vi "InitCursor.vi"(8 "error in (no error)":errorcluster, 11 "Menu in":refnum<class "Menu.lvclass">) -> (0 "error out":errorcluster, 3 "Menu out":refnum<class "Menu.lvclass">)   [LabVIEW 2019, in "RT_Game.lvlib" / "Menu.lvclass"]
uses:
  Menu.lvclass
  C:/Users/FreshBob/Dropbox/VIs/myRIO_GameConsole/RT/RT_Game/Game/Game.lvclass
  Cursor/Cursor.lvclass
  C:/Users/FreshBob/Dropbox/VIs/myRIO_GameConsole/RT/RT_Game/GameObject/GameObject.lvclass
  C:/Users/FreshBob/Dropbox/VIs/myRIO_GameConsole/RT/RT_Game/RT_Sprite/RT_Sprite.lvclass
  Game/Coordinate.ctl
  Menu.lvclass/Menu.ctl
  Cursor/Cursor.lvclass/Cursor.ctl
  GameObject/GameObject.lvclass/GameObject.ctl
  Game/Game.lvclass/Game.ctl
  Cursor/Write Positions.vi
  Cursor/Write selection.vi
  Cursor/Write speed.vi
  GameObject/Write IsActive.vi
  Cursor/Write Wrap.vi
  Game/Write Sprite1.vi
  Game/Game.lvclass
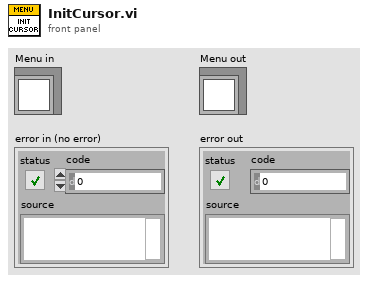
[diagram p1: front panel]
types:
  T1 = typedef "RT_Game.lvlib/Game.lvclass/Coordinate.ctl" = cluster{"x":dbl, "y":dbl}
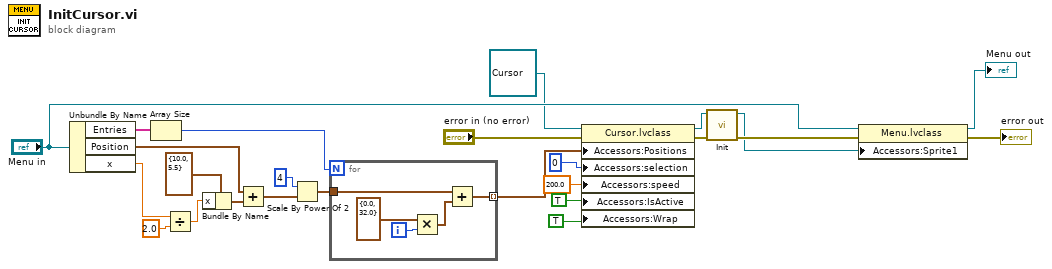
[diagram p0: block diagram]
diagram:
  n1 = Unbundle By Name("Menu in") -> ("Entries"=w10:string[], "Position"=w11:T1, "x"=w14:dbl)
  n2 = Array Size(array=w10) -> (size(s)=w18:i32)
  n3 = Divide(x=w14, y=2.0) -> (x/y=w16:dbl)
  n4 = Bundle By Name(cluster=T1 {"x"=10.0, "y"=5.5} ("y"), "x"=w16) -> (w13:T1)
  n5 = Add(x=w11, y=w13) -> (x+y=w17:T1)
  n6 = Scale By Power Of 2(n=i16 4, x=w17) -> (x*2^n=w19:T1)
  n7 = for {
    N: w18 -> [_]
    tunnel: w19 -> [w29]
    tunnel: [w26] -> w21 mode=indexing
    i -> [w30]
    n8 = Multiply(x=T1 {"x"=0.0, "y"=32.0} ("Position"), y=w30) -> (x*y=w27:T1)
    n9 = Add(x=w29, y=w27) -> (x+y=w26:T1)
  }
  n10 = property class="Cursor.lvclass"(reference=refnum<class "Cursor.lvclass"> refnum ("RT_Game.lvlib:Cursor.lvclass"), error in="error in (no error)", "Accessors:Positions"=w21, "Accessors:selection"=i16 0 ("selection"), "Accessors:speed"=200.0 ("speed"), "Accessors:IsActive"=TRUE ("IsActive"), "Accessors:Wrap"=TRUE ("Wrap")) -> (reference out=w7:refnum<class "Cursor.lvclass">, error out=w8:errorcluster)
  n11 = call-dynamic "Init.vi"("error in (no error)"=w8, "Cursor in"=w7) -> ("error out"=w25:errorcluster, "Cursor out"=w3:refnum<class "Cursor.lvclass">)  [unwired: 8 in]
  n12 = property class="Menu.lvclass"(reference="Menu in", error in=w25, "Accessors:Sprite1"=w3) -> (reference out=→"Menu out":refnum<class "Menu.lvclass">, error out=→"error out":errorcluster)
